vi "Add devices to expt line menu.vi"(8 "error in (no error)":errorcluster, 9 "All Devices":string[](array[string]), 10 "menu reference":refnum<k9>, 11 "This vi ref":refnum<vi>) -> (0 "error out":errorcluster)   [LabVIEW 2013]
panel:
  out "Expt_Line":string
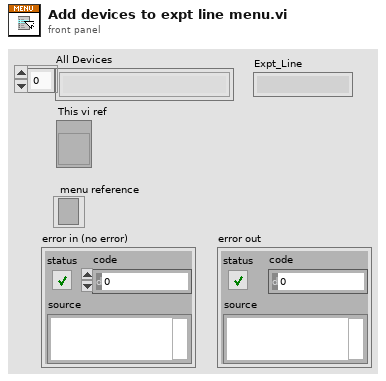
[diagram p1: front panel]
types:
  T1 = typedef "mysql_authentication.ctl" = cluster{"User":string, "Password":string, "Database":string}
  T2 = cluster{"Port":u16, "IP Address":string, "Authentication":T1}
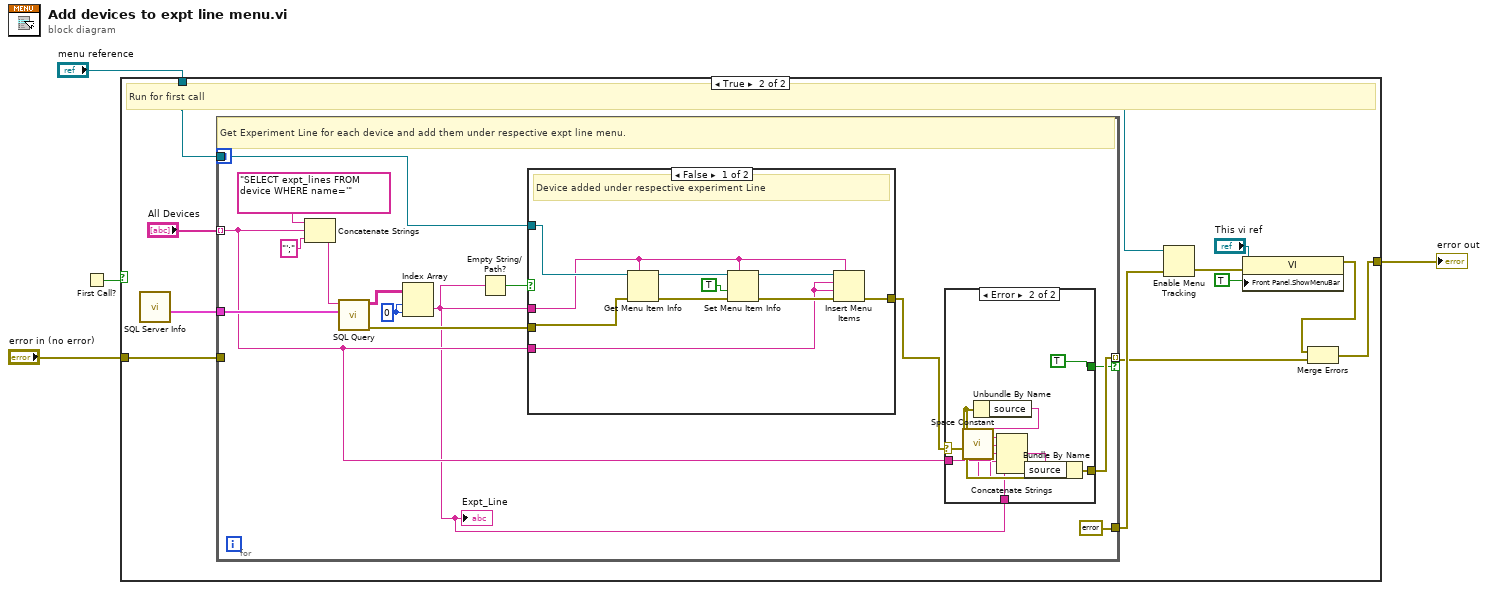
[diagram p0: block diagram]
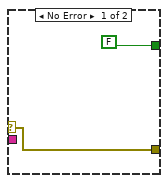
[diagram p3: hidden frame]
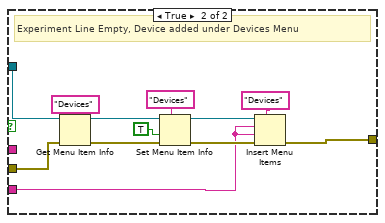
[diagram p4: hidden frame]
diagram:
  n1 = First Call?() -> (First Call?: T/F=w1:bool)
  n2 = case shown="True" w1 {
    tunnel: "error in (no error)" -> [w5 w16]
    tunnel: "menu reference" -> [_ w15]
    tunnel: [w5 w6] -> w2
    frame False {
    }
    frame True {
      # "Run for first call"
      n3 = call "SQL Server Info.vi"() -> ("SQL Server Info"=w10:T2)
      n4 = for {
        tunnel: w10 -> [w28]
        tunnel: "All Devices" -> [w21] mode=indexing
        tunnel: w15 -> [w24]
        tunnel: w16 -> [_]
        tunnel: [w19] -> w7 mode=indexing if=w17
        tunnel: [errorcluster {"status"=FALSE, "code"=0, "source"=""} ("error in (no error)")] -> w9
        w27 = 0 ("disabled index (col)")
        # "Get Experiment Line for each device and add them under respective expt line menu."
        n5 = Concatenate Strings("SELECT expt_lines FROM device WHERE name='" ("Query"), w21, "';" ("string")) -> (w22:string)
        n6 = call "SQL Query.vi"("SQL Server Info"=w28, "Query"=w22) -> ("error out"=w26:errorcluster, "data"=w31:string[][])  [unwired: 8 in]
        n7 = Index Array(array=w31, index (row)=w27, index (col)=w27) -> (element=w20:string)
        "Expt_Line" <- w20
        n8 = Empty String/Path?(string/path=w20) -> (empty?=w25:bool)
        n9 = case shown="False" w25 {
          tunnel: [w42 w52] -> w18
          tunnel: w26 -> [w46 w58]
          tunnel: w21 -> [w45 w57]
          tunnel: w24 -> [w44 w56]
          tunnel: w20 -> [w43 _]
          frame False {
            # "Device added under respective experiment Line"
            n10 = Get Menu Item Info(7:w43, 8:w46, 11:w44) -> (0:w47:errorcluster, 3:w51:refnum<k9>)  [unwired: 5 out]
            n11 = Set Menu Item Info(7:w43, 8:w47, 9:TRUE ("enabled"), 11:w51) -> (0:w48:errorcluster, 3:w49:refnum<k9>)  [unwired: 3 in]
            n12 = Insert Menu Items(5:w43, 6:w48, 7:w45, 8:w45, 9:w49) -> (0:w42:errorcluster)  [unwired: 1 in, 2 out]
          }
          frame True {
            # "Experiment Line Empty, Device added under Devices Menu"
            n13 = Get Menu Item Info(7:"Devices", 8:w58, 11:w56) -> (0:w59:errorcluster, 3:w63:refnum<k9>)  [unwired: 5 out]
            n14 = Set Menu Item Info(7:"Devices", 8:w59, 9:TRUE ("enabled"), 11:w63) -> (0:w60:errorcluster, 3:w61:refnum<k9>)  [unwired: 3 in]
            n15 = Insert Menu Items(5:"Devices" ("menu tag"), 6:w60, 7:w57, 8:w57, 9:w61) -> (0:w52:errorcluster)  [unwired: 1 in, 2 out]
          }
        }
        n16 = case shown="Error" w18 {
          selector: w18 -> [w33 w41]
          tunnel: w21 -> [_ w38]
          tunnel: w20 -> [_ w37]
          tunnel: [w33 w35] -> w19
          tunnel: [FALSE TRUE] -> w17
          frame No Error {
          }
          frame Error {
            n17 = call <vilib>:"Space Constant.vi"() -> ("String"=w36:string)
            n18 = Unbundle By Name(w41) -> ("source"=w40:string)
            n19 = Concatenate Strings(w40, w36, w38, w36, w37) -> (w39:string)
            n20 = Bundle By Name(cluster=w41, "source"=w39) -> (w35:errorcluster)
          }
        }
      }
      n21 = Enable Menu Tracking(2:w9, 4:w15) -> (0:w13:errorcluster)  [unwired: 1 in, 1 out]
      n22 = property class="VI"(reference="This vi ref", error in=w13, "Front Panel.ShowMenuBar"=TRUE ("Edit Mode On Open")) -> (error out=w8:errorcluster)  [unwired: 1 out]
      n23 = Merge Errors(w8, w7) -> (w6:errorcluster)
    }
  }
  "error out" <- w2
